vi "Custom_AND.vi"(8 "Input B":bool, 11 "Input A":bool) -> (3 "Output Y":bool)   [LabVIEW 2026]
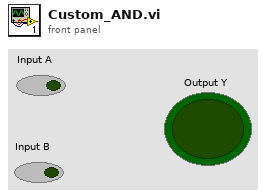
[diagram p1: front panel]
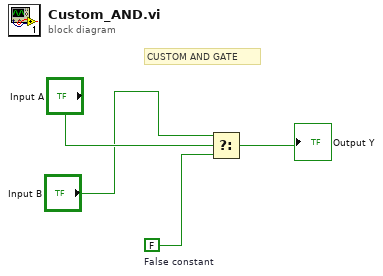
[diagram p0: block diagram]
diagram:
  w3 = FALSE  # False constant
  # "CUSTOM AND GATE"
  n1 = Select(t="Input B", s="Input A", f=w3) -> (s? t:f=→"Output Y":bool)
